vi "Get Basic Info.vi"(5 "교정정보 in":T1, 6 "출장교정 List":refnum<vi>, 7 "등록번호":string, 8 "에러 입력(에러 없음)":errorcluster, 10 "현장리스트?":bool, 11 "참조 번호 입력":T2) -> (0 "에러 출력":errorcluster, 1 "None?":bool, 2 "교정정보 out":T1, 3 "참조 번호 출력":T2, 4 "기타정보":string[](array[string]))   [LabVIEW 2020]
uses:
  Controls/Clst_Cal Info Global.ctl
  <vilib>/addons/database/Connection.llb/Conn ObjectReference.ctl
  Controls/Cmd_Read Query.ctl
  Controls/Clst_Query Info.ctl
  Variables/Global_Cal Info.vi
  <vilib>/addons/database/NI_Database_API.lvlib
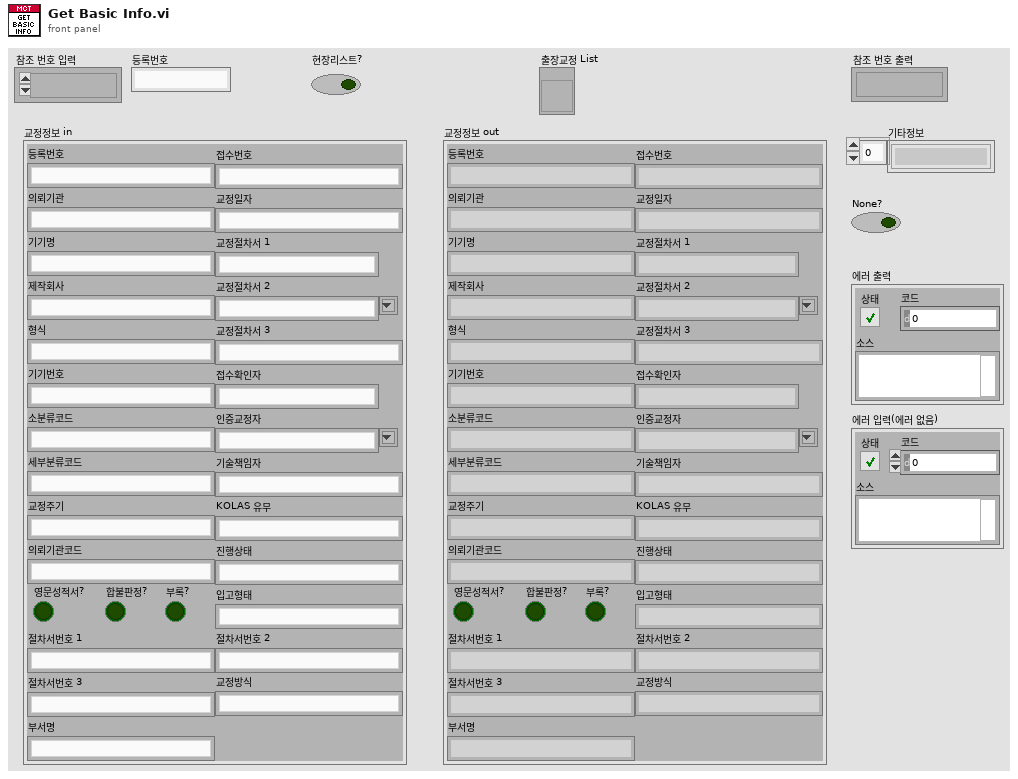
[diagram p1: front panel]
types:
  T1 = typedef "Clst_Cal Info Global.ctl" = cluster{"등록번호":string, "의뢰기관":string, "기기명":string, "제작회사":string, "형식":string, "기기번호":string, "소분류코드":string, "세부분류코드":string, "교정주기":string, "접수번호":string, "교정일자":string, "교정절차서 1":string, "교정절차서 2":string, "교정절차서 3":string, "접수확인자":string, "인증교정자":string, "기술책임자":string, "KOLAS 유무":string, "진행상태":string, "의뢰기관코드":string, "입고형태":string, "영문성적서?":bool, "합불판정?":bool, "부록?":bool, "절차서번호 1":string, "절차서번호 2":string, "절차서번호 3":string, "교정방식":string, "부서명":string}
  T2 = typedef "NI_Database_API.lvlib/Conn ObjectReference.ctl" = refnum<k1>
  T3 = typedef "Clst_Query Info.ctl" = cluster{"사번":string, "등록번호":string, "업체명":string, "세부분류코드":string, "형식":string, "기기번호":string, "FUNC":string, "FUNC_EXT":string, "옵션":string, "추가문자열":string, "일자":string, "배열 1":string[], "배열 2":string[], "항목명":string, "문자열":string, "이름":string}
  T4 = typedef "Cmd_Read Query.ctl" = enum16{"교정자 이름 얻기", "인증교정자 얻기", "기술책임자 얻기", "기책부책 얻기", "등록번호 얻기", "등록정보 얻기", "업체정보 얻기", "교정일자(CAMAS) 얻기", "교정일자(CALSTD) 얻기", "교정환경 얻기", "교정절차서 목록 얻기", "교정절차서명 얻기", "교정절차 목록얻기", "교정절차 얻기", "PROC 교정절차 얻기", "PROC SPEC 얻기", "교정절차(Func별) 얻기", "교정절차(Func_ext별) 얻기", "기관코드 얻기", "교정기능(세부분류) 얻기", "교정기능(모델) 얻기", "교정기능 목록 얻기", "교정기능 명칭 얻기", "교정기능 항목명칭 얻기", "DB (사용기준기) 얻기", "DB (기준기이름) 얻기", "DB (기준기이름목록) 얻기", "DB (기준기목록) 얻기", "DB (기준기값) 얻기", "DB (CMC) 얻기", "DB (FUNC) 얻기", "DB (CALNAME) 얻기", "DB (STDNAME) 얻기", "DB (SPEC) 얻기", "모델(항목전체) 얻기", "모델(최대범위) 얻기", "모델(최소범위) 얻기", "모델(최대최소) 얻기", "모델(범위조건) 얻기", "모델(등록요청) 얻기", "모델(형식별) 얻기", "모델(조건별) 얻기", "모델(모델검색) 얻기", "세부분류 목록 얻기", "기준기등록리스트 얻기", "STD Cal Date Check", "DB등록일자 얻기", "적용항목 얻기", "기타정보 얻기", "기준기요청 얻기", "서버버전 얻기"}
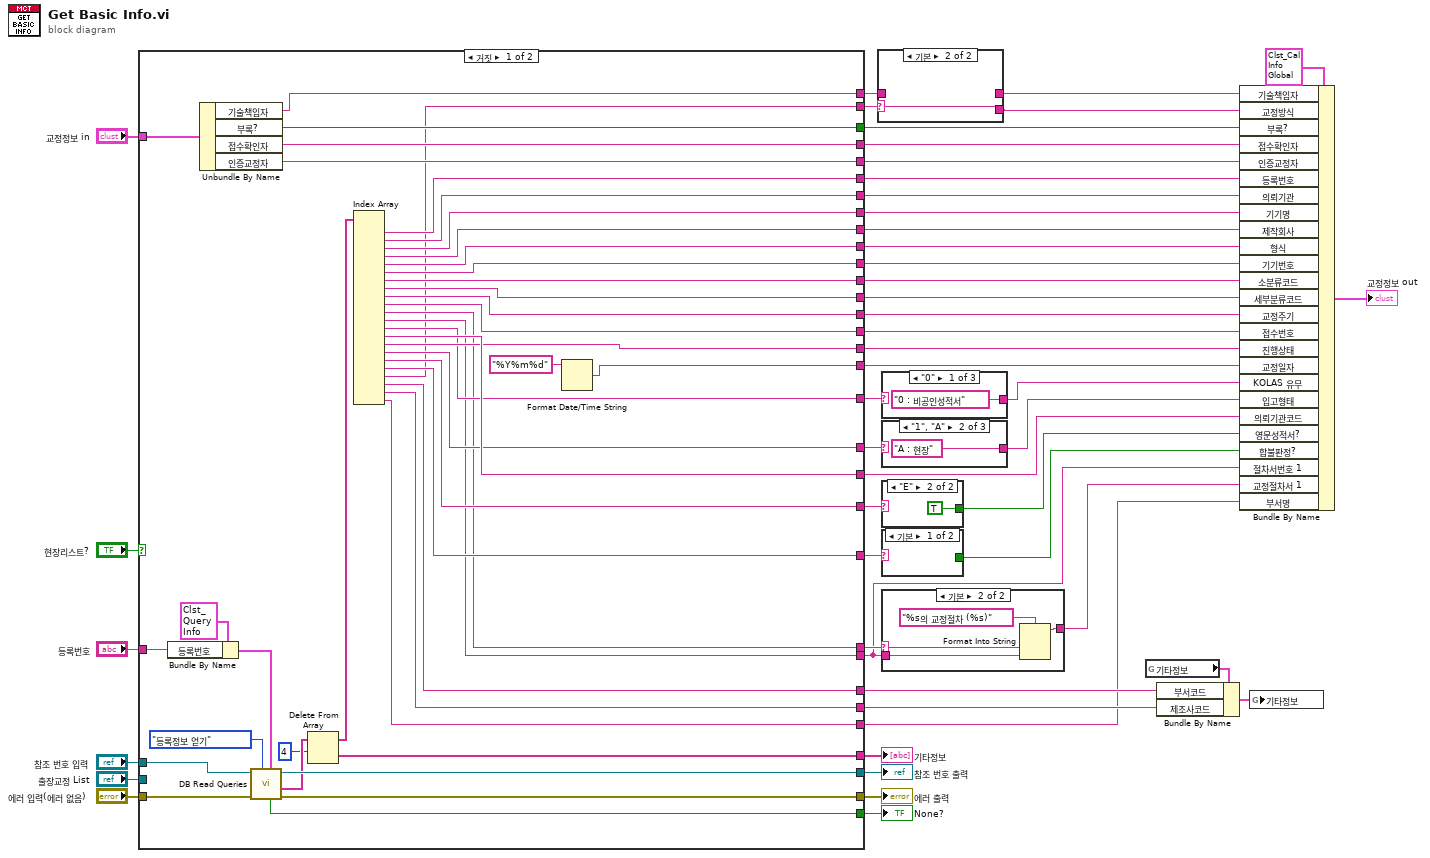
[diagram p0: block diagram]
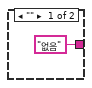
[diagram p3: hidden frame]
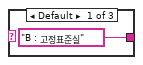
[diagram p4: hidden frame]
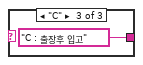
[diagram p5: hidden frame]
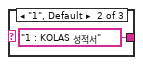
[diagram p6: hidden frame]
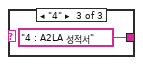
[diagram p7: hidden frame]
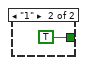
[diagram p8: hidden frame]
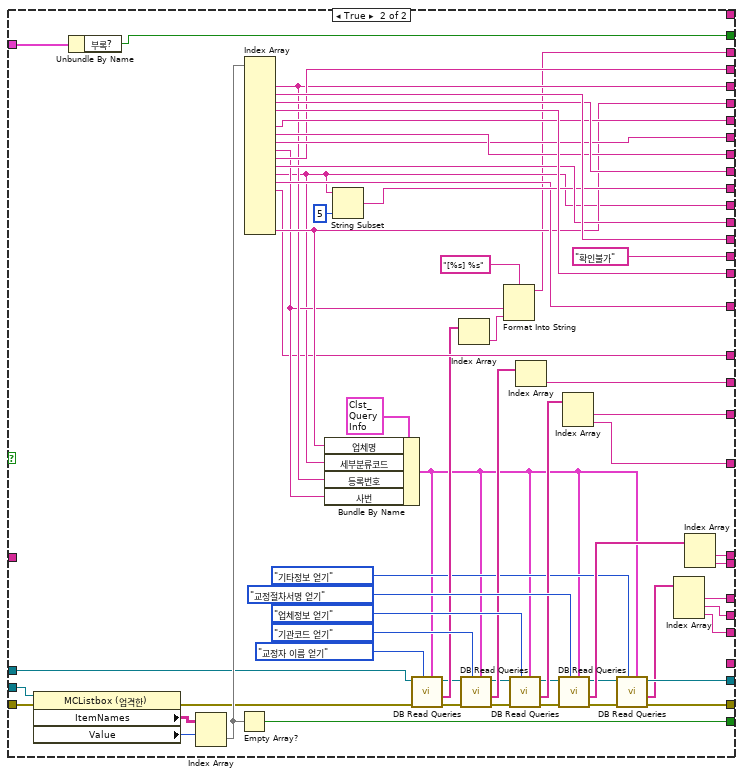
[diagram p10: hidden frame]
diagram:
  n1 = case shown="거짓" "현장리스트?" {
    tunnel: [w63 w134] -> w21
    tunnel: [w65 w146] -> w47
    tunnel: "에러 입력(에러 없음)" -> [w90 w150]
    tunnel: "참조 번호 입력" -> [w89 w101]
    tunnel: [w88 w98] -> w44
    tunnel: "등록번호" -> [w87 _]
    tunnel: [w86 w127] -> w14
    tunnel: [w85 w131] -> w41
    tunnel: [w84 w141] -> w40
    tunnel: [w83 w139] -> w39
    tunnel: [w82 w140] -> w38
    tunnel: [w81 w142] -> w37
    tunnel: [w80 w136] -> w36
    tunnel: [w79 w118] -> w35
    tunnel: [w78 w137] -> w34
    tunnel: [w77 w144] -> w33
    tunnel: [w76 w130] -> w10
    tunnel: [w75 "확인불가" ("문자열")] -> w32
    tunnel: [w74 w97] -> w31
    tunnel: "출장교정 List" -> [_ w149]
    tunnel: [w69 w143] -> w28
    tunnel: [w68 w138] -> w13
    tunnel: [w67 w122] -> w27
    tunnel: [w66 w121] -> w26
    tunnel: [w57 w116] -> w19
    tunnel: "교정정보 in" -> [w64 w117]
    tunnel: [w59 _] -> w22
    tunnel: [w62 w113] -> w20
    tunnel: [w56 w112] -> w18
    tunnel: [w55 w111] -> w17
    tunnel: [w54 w110] -> w15
    tunnel: [w53 _] -> w9
    tunnel: [w52 _] -> w7
    tunnel: [w51 w93] -> w4
    tunnel: [w50 w92] -> w3
    tunnel: [w49 w91] -> w1
    frame False {
      n2 = Bundle By Name(cluster=T3 {"사번"="", "등록번호"="", "업체명"="", "세부분류코드"="", "형식"="", "기기번호"="", "FUNC"="", "FUNC_EXT"="", "옵션"="", "추가문자열"="", "일자"="", "배열 1"=[], "배열 2"=[], "항목명"="", "문자열"="", "이름"=""} ("Query info"), "등록번호"=w87) -> (w71:T3)
      n3 = Unbundle By Name(w64) -> ("기술책임자"=w52:string, "부록?"=w57:bool, "접수확인자"=w56:string, "인증교정자"=w68:string)
      n4 = call "DB Read Queries.vi"("Query info"=w71, "Query Command"=Cmd_Read_Query."등록정보 얻기", "에러 입력(에러 없음)"=w90, "참조 번호 입력"=w89) -> ("에러 출력"=w74:errorcluster, "Data (0번행)"=w61:string[], "참조 번호 출력"=w88:T2, "None?"=w65:bool)  [unwired: 3 in, 1 out]
      n5 = Delete From Array(array=w61, length=4 ("길이")) -> (deleted portion=w59:string[], array with subset deleted=w58:string[])  [unwired: 1 in]
      n6 = Index Array(array=w58) -> (element #1=w86:string, element #2=w85:string, element #3=w84:string, element #4=w83:string, element #5=w82:string, element #6=w81:string, element #7=w80:string, element #8=w79:string, element #9=w78:string, element #10=w77:string, element #11=w55:string, element #12=w54:string, element #13=w63:string, element #14=w76:string, element #15=w75:string, element #16=w62:string, element #17=w67:string, element #18=w66:string, element #19=w53:string, element #20=w51:string, element #21=w50:string, element #22=w49:string)  [unwired: 22 in]
      n7 = Format Date/Time String(time format string (%c)="%Y%m%d" ("시간 포맷 문자열 (%c)")) -> (date/time string=w69:string)  [unwired: 2 in]
    }
    frame True {
      n8 = property class="MCListbox (엄격한)"(reference=w149, error in=w150) -> (error out=w102:errorcluster, "ItemNames"=w148:string[][], "Value"=w147:i32)  [unwired: 1 out]
      n9 = Unbundle By Name(w117) -> ("부록?"=w116:bool)
      n10 = Index Array(array=w148, index (row)=w147) -> (element=w145:string[])  [unwired: 1 in]
      n11 = Empty Array?(array=w145) -> (empty?=w146:bool)
      n12 = Index Array(array=w145) -> (element #2=w127:string, element #3=w144:string, element #4=w142:string, element #5=w143:string, element #7=w141:string, element #8=w140:string, element #9=w139:string, element #10=w123:string, element #11=w138:string, element #12=w137:string, element #13=w118:string, element #14=w134:string, element #15=w113:string, element #20=w131:string)  [unwired: 20 in, 6 out]
      n13 = Bundle By Name(cluster=T3 {"사번"="", "등록번호"="", "업체명"="", "세부분류코드"="", "형식"="", "기기번호"="", "FUNC"="", "FUNC_EXT"="", "옵션"="", "추가문자열"="", "일자"="", "배열 1"=[], "배열 2"=[], "항목명"="", "문자열"="", "이름"=""} ("Query info"), "업체명"=w131, "세부분류코드"=w118, "등록번호"=w127, "사번"=w123) -> (w95:T3)
      n14 = String Subset(string=w118, length (rest)=5 ("길이(나머지)")) -> (substring=w136:string)  [unwired: 1 in]
      n15 = call "DB Read Queries.vi"("Query info"=w95, "Query Command"=Cmd_Read_Query."교정자 이름 얻기", "에러 입력(에러 없음)"=w102, "참조 번호 입력"=w101) -> ("에러 출력"=w103:errorcluster, "Data (0번행)"=w109:string[], "참조 번호 출력"=w104:T2)  [unwired: 3 in, 2 out]
      n16 = Index Array(array=w109) -> (element=w125:string)  [unwired: 1 in]
      n17 = call "DB Read Queries.vi"("Query info"=w95, "Query Command"=Cmd_Read_Query."기관코드 얻기", "에러 입력(에러 없음)"=w103, "참조 번호 입력"=w104) -> ("에러 출력"=w106:errorcluster, "Data (0번행)"=w119:string[], "참조 번호 출력"=w105:T2)  [unwired: 3 in, 2 out]
      n18 = Format Into String(format string="[%s] %s" ("포맷 문자열"), w123, w125) -> (resulting string=w112:string)  [unwired: 2 in, 1 out]
      n19 = call "DB Read Queries.vi"("Query info"=w95, "Query Command"=Cmd_Read_Query."업체정보 얻기", "에러 입력(에러 없음)"=w106, "참조 번호 입력"=w105) -> ("에러 출력"=w107:errorcluster, "Data (0번행)"=w115:string[], "참조 번호 출력"=w108:T2)  [unwired: 3 in, 2 out]
      n20 = Index Array(array=w119) -> (element=w130:string)  [unwired: 1 in]
      n21 = call "DB Read Queries.vi"("Query info"=w95, "Query Command"=Cmd_Read_Query."교정절차서명 얻기", "에러 입력(에러 없음)"=w107, "참조 번호 입력"=w108) -> ("에러 출력"=w99:errorcluster, "Data (0번행)"=w120:string[], "참조 번호 출력"=w100:T2)  [unwired: 3 in, 2 out]
      n22 = Index Array(array=w115) -> (element #1=w122:string, element #2=w121:string)  [unwired: 2 in]
      n23 = call "DB Read Queries.vi"("Query info"=w95, "Query Command"=Cmd_Read_Query."기타정보 얻기", "에러 입력(에러 없음)"=w99, "참조 번호 입력"=w100) -> ("에러 출력"=w97:errorcluster, "Data (0번행)"=w94:string[], "참조 번호 출력"=w98:T2)  [unwired: 3 in, 2 out]
      n24 = Index Array(array=w94) -> (element #1=w93:string, element #2=w92:string, element #3=w91:string)  [unwired: 3 in]
      n25 = Index Array(array=w120) -> (element #1=w111:string, element #2=w110:string)  [unwired: 2 in]
    }
  }
  "None?" <- w47
  "에러 출력" <- w31
  "참조 번호 출력" <- w44
  "기타정보" <- w22
  n26 = case shown="기본" w9 {
    selector: w9 -> [w151 w153]
    tunnel: [w152 _] -> w8
    tunnel: w7 -> [w152 _]
    tunnel: [w151 w153] -> w6
    frame "02" {
    }
    frame Default {
    }
  }
  n27 = case shown="\"0\"" w21 {
    tunnel: ["0 : 비공인성적서" "1 : KOLAS 성적서" "4 : A2LA 성적서"] -> w12
    frame "0" {
    }
    frame "1", Default {
    }
    frame "4" {
    }
  }
  n28 = case shown="\"1\", \"A\"" w20 {
    tunnel: ["B : 고정표준실" "A : 현장" "C : 출장후 입고"] -> w11
    frame Default {
    }
    frame "1", "A" {
    }
    frame "C" {
    }
  }
  n29 = case shown="\"E\"" w27 {
    tunnel: [_ TRUE] -> w25
    frame Default {
    }
    frame "E" {
    }
  }
  n30 = case shown="기본" w26 {
    tunnel: [_ TRUE] -> w24
    frame Default {
    }
    frame "1" {
    }
  }
  n31 = case shown="기본" w17 {
    selector: w17 -> [_ w163]
    tunnel: w15 -> [_ w165]
    tunnel: ["없음" w164] -> w16
    frame "" {
    }
    frame Default {
      n32 = Format Into String(format string="%s의 교정절차 (%s)" ("포맷 문자열"), w163, w165) -> (resulting string=w164:string)  [unwired: 2 in, 1 out]
    }
  }
  n33 = global read "Global_Cal Info.vi" "기타정보"() -> (w5:cluster{"부서코드":string, "제조사코드":string})
  n34 = Bundle By Name(cluster=w5, "부서코드"=w4, "제조사코드"=w3) -> (w2:cluster{"부서코드":string, "제조사코드":string})
  n35 = Bundle By Name(cluster=T1 {"등록번호"="", "의뢰기관"="", "기기명"="", "제작회사"="", "형식"="", "기기번호"="", "소분류코드"="", "세부분류코드"="", "교정주기"="", "접수번호"="", "교정일자"="", "교정절차서 1"="", "교정절차서 2"="", "교정절차서 3"="", "접수확인자"="", "인증교정자"="", "기술책임자"="", "KOLAS 유무"="", "진행상태"="", "의뢰기관코드"="", "입고형태"="", "영문성적서?"=FALSE, "합불판정?"=FALSE, "부록?"=FALSE, "절차서번호 1"="", "절차서번호 2"="", "절차서번호 3"="", "교정방식"="", "부서명"=""} ("교정정보"), "기술책임자"=w8, "교정방식"=w6, "부록?"=w19, "접수확인자"=w18, "인증교정자"=w13, "등록번호"=w14, "의뢰기관"=w41, "기기명"=w40, "제작회사"=w39, "형식"=w38, "기기번호"=w37, "소분류코드"=w36, "세부분류코드"=w35, "교정주기"=w34, "접수번호"=w33, "진행상태"=w32, "교정일자"=w28, "KOLAS 유무"=w12, "입고형태"=w11, "의뢰기관코드"=w10, "영문성적서?"=w25, "합불판정?"=w24, "절차서번호 1"=w15, "교정절차서 1"=w16, "부서명"=w1) -> (→"교정정보 out":T1)
  n36 = global write "Global_Cal Info.vi" "기타정보"(w2) -> ()
